vi "grub.vi"() -> ()   [LabVIEW 2014]
uses:
  <instrlib>/niDMM/nidmm.llb/niDMM Waveform Function.ctl
  <vilib>/Analysis/3filter.llb/Filter Passband Type.ctl
  <vilib>/Waveform/WDTOps.llb/WDT Get Waveform Subset DBL.vi
  <vilib>/Analysis/baseanly.llb/IIR Cascade Filter (DBL).vi
  <instrlib>/niDMM/nidmm.llb/niDMM Read Waveform (waveform data).vi
  <vilib>/Analysis/NI_AALBase.lvlib
  <vilib>/measure/NI_MABase.lvlib
  <vilib>/Analysis/NI_AALPro.lvlib
panel:
  in  "high cutoff freq: fh":dbl=0.45 format="%#_13g"
  out "DC estimate (V)":dbl caption="直流分量估计(V)" format="%0.2f"
  out "元素":waveform(dbl)
  in  "order":i32=2 caption="阶数"
  in  "low cutoff freq: fl":dbl=0.12500000000000006 caption="低截止频率:fl" format="%0.4f"
  out "波形图":ext[][](graph)
  out "Actual Number":i32
  in  "停止":bool
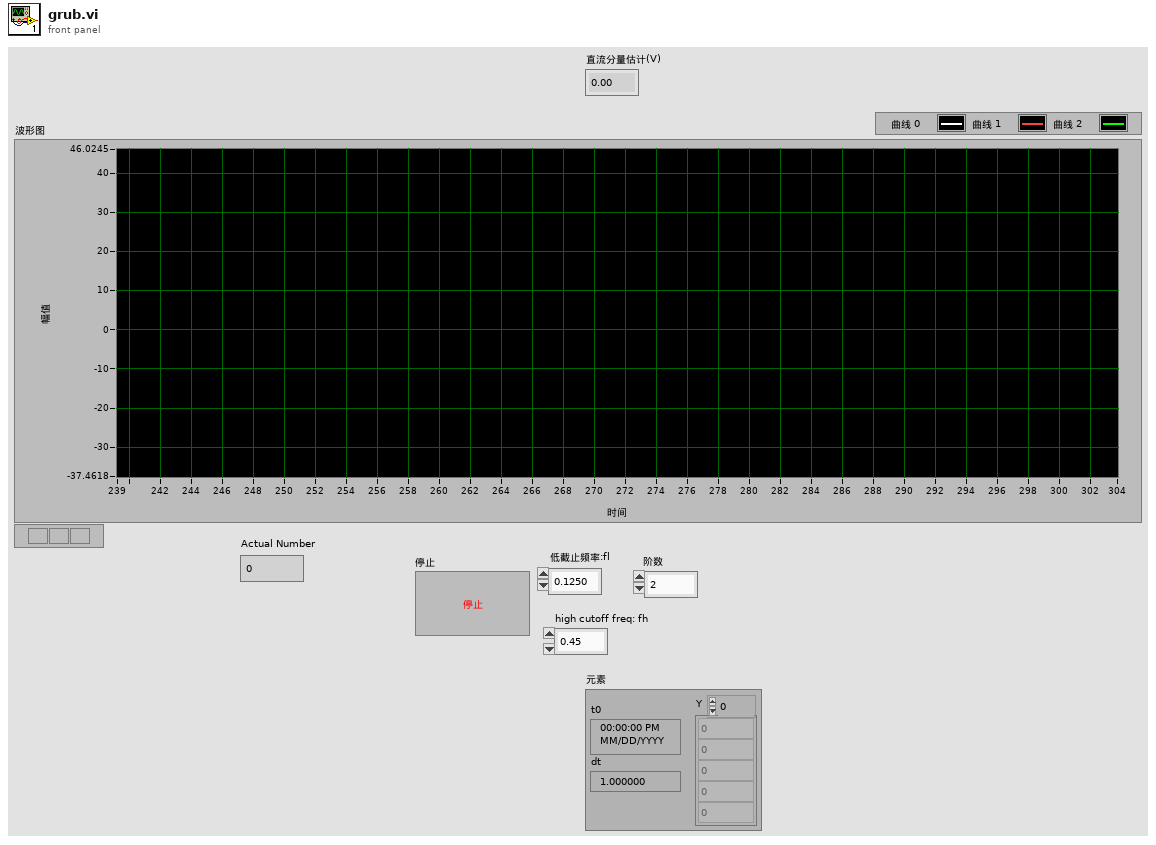
[diagram p1: front panel]
types:
  T1 = typedef "niDMM Waveform Function.ctl" = i32
  T2 = typedef "NI_AALBase.lvlib/Filter Passband Type.ctl" = enum32{"Lowpass", "Highpass", "Bandpass", "Bandstop"}
  T3 = cluster{"filter structure":enum32{"IIR 2nd Order", "IIR 4th Order"}, "Reverse Coefficients":dbl[], "Forward Coefficients":dbl[]}
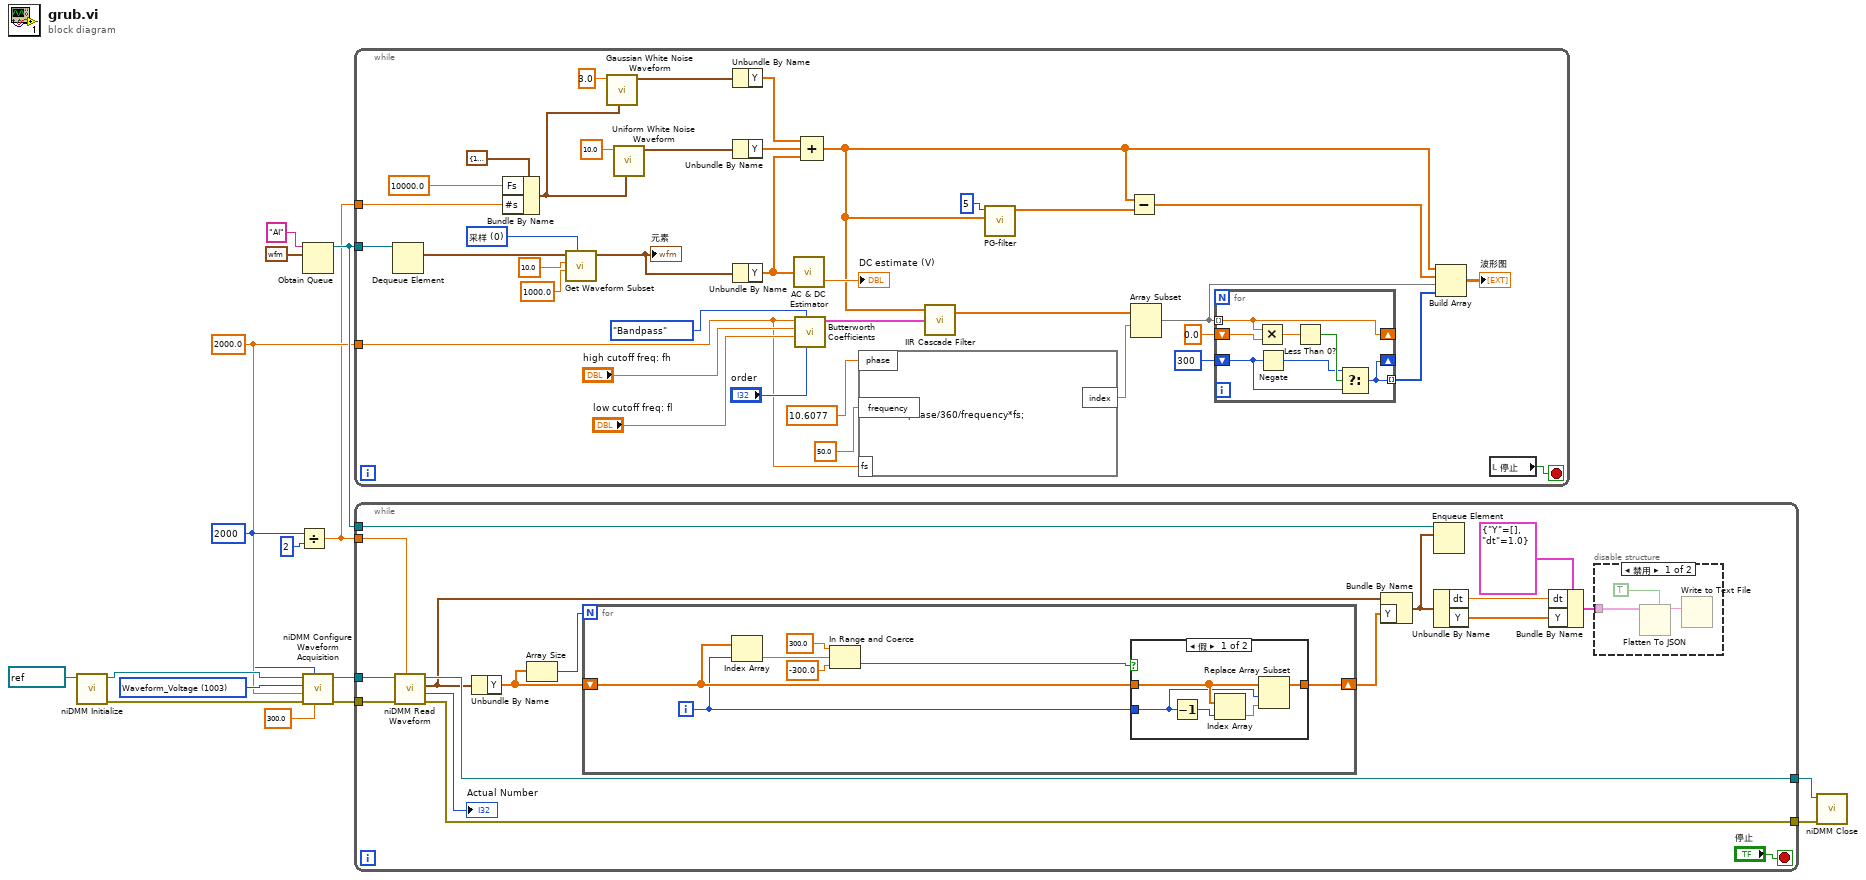
[diagram p0: block diagram]
diagram:
  w2 = 2000 ("Waveform Points")
  w4 = 2000.0 ("Rate")
  w16 = T1 1003 items=["Waveform_Voltage"=1003, "Waveform_Current"=1004] ("Function")
  n1 = call <instrlib>:"niDMM Initialize.vi"("Instrument Descriptor"=refnum<k15> "Dev1" ("instrument handle")) -> ("error out"=w13:errorcluster, "instrument handle out"=w14:refnum<k15>)  [unwired: 9 in]
  n2 = Divide(x=w2, y=2) -> (x/y=w1:dbl)
  n3 = Obtain Queue(name (unnamed)="AI" ("名称（未命名）"), element data type=waveform(dbl) {"t0"=timestamp(0 s since 1904-01-01), "dt"=1.0, "Y"=[]} ("输出波形")) -> (queue out=w5:refnum<queue>)  [unwired: 3 in, 2 out]
  n4 = call <instrlib>:"niDMM Configure Waveform Acquisition.vi"("Range"=300.0, "Waveform Points"=w2, "error in (no error)"=w13, "Rate"=w4, "Function"=w16, "instrument handle"=w14) -> ("error out"=w10:errorcluster, "instrument handle out"=w11:refnum<k15>)  [unwired: 4 in]
  n5 = while {
    tunnel: w5 -> [w53]
    tunnel: w4 -> [w22]
    tunnel: w1 -> [w43]
    stop <- w54 stop-if-true
    w30 = u16 0 items=["采样", "相对时间"] ("start/duration format")
    n6 = Dequeue Element(queue=w53) -> (element=w42:waveform(dbl))  [unwired: 2 in, 3 out]
    n7 = Bundle By Name(cluster=cluster{"Fs":dbl, "#s":dbl} {"Fs"=1000.0, "#s"=1000.0} ("sampling info"), "Fs"=10000.0, "#s"=w43) -> (w35:cluster{"Fs":dbl, "#s":dbl})
    n8 = call-poly <vilib>:"Get Waveform Subset.vi"("start/duration format"=w30, "duration"=1000.0, "start samples/time"=10.0, "waveform in"=w42) -> ("waveform out"=w32:waveform(dbl))  [unwired: 2 in, 3 out]
    "元素" <- w32
    n9 = call <vilib>:"Gaussian White Noise Waveform.vi"("sampling info"=w35, "standard deviation"=3.0) -> ("signal out"=w38:waveform(dbl))  [unwired: 8 in, 1 out]
    n10 = call <vilib>:"Uniform White Noise Waveform.vi"("sampling info"=w35, "amplitude"=10.0) -> ("signal out"=w41:waveform(dbl))  [unwired: 8 in, 1 out]
    n11 = Unbundle By Name(w38) -> ("Y"=w37:dbl[])
    n12 = Unbundle By Name(w41) -> ("Y"=w40:dbl[])
    n13 = Unbundle By Name(w32) -> ("Y"=w34:dbl[])
    n14 = call <vilib>:"AC & DC Estimator.vi"("Signal (V)"=w34) -> ("DC estimate (V)"=→"DC estimate (V)":dbl)  [unwired: 1 out]
    n15 = call <vilib>:"Butterworth Coefficients.vi"("order"="order", "filter type"=Filter_Passband_Type."Bandpass", "low cutoff freq: fl"="low cutoff freq: fl", "high cutoff freq: fh"="high cutoff freq: fh", "sampling freq: fs"=w22) -> ("IIR Filter Cluster"=w26:T3)  [unwired: 5 in, 1 out]
    n16 = Compound Arithmetic op=ADD(w37, w40, w34) -> (w27:dbl[])
    n17 = formula code="index = phase/360/frequency*fs;"("phase"=10.6077, "frequency"=50.0 ("输入变量"), "fs"=w22) -> ("index"=w21:dbl)
    n18 = call-poly <vilib>:"IIR Cascade Filter.vi"("IIR Filter Cluster"=w26, "X"=w27) -> ("Filtered X"=w25:dbl[])  [unwired: 1 in, 1 out]
    n19 = call "PG-filter.vi"("Y"=w27, "n"=i16 5) -> ("数组"=w52:ext[])  [unwired: 9 in]
    n20 = Subtract(x=w27, y=w52) -> (x-y=w49:ext[])
    n21 = Array Subset(array=w25, index=w21) -> (w20:dbl[])  [unwired: 1 in]
    n22 = for {
      tunnel: w20 -> [w59] mode=indexing
      shift-right: [w59] -> _
      shift-left: 0.0 -> [w61]
      shift-right: [w56] -> _
      shift-left: 300 -> [w57]
      tunnel: [w56] -> w17 mode=indexing
      n23 = Multiply(x=w59, y=w61) -> (x*y=w60:dbl)
      n24 = Negate(x=w57) -> (-x=w55:i32)
      n25 = Less Than 0?(x=w60) -> (x < 0?=w58:bool)
      n26 = Select(t=w55, s=w58, f=w57) -> (s? t:f=w56:i32)
    }
    n27 = Build Array(w27, w49, w20, w17) -> (→"波形图":ext[][])
    n28 = local read "停止"() -> (w54:bool)
  }
  n29 = while {
    tunnel: w11 -> [w78]
    tunnel: w10 -> [w77]
    tunnel: [w76] -> w9
    tunnel: [w75] -> w8
    tunnel: w5 -> [w64]
    tunnel: w1 -> [w62]
    stop <- "停止" stop-if-true
    n30 = call-poly <instrlib>:"niDMM Read Waveform.vi"("Number To Read"=w62, "error in (no error)"=w77, "instrument handle"=w78) -> ("error out"=w75:errorcluster, "Actual Number"=→"Actual Number":i32, "Waveform Data"=w73:waveform(dbl), "instrument handle out"=w76:refnum<k15>)  [unwired: 5 in]
    n31 = Unbundle By Name(w73) -> ("Y"=w71:dbl[])
    n32 = Array Size(array=w71) -> (size(s)=w70:i32)
    n33 = for {
      N: w70 -> [_]
      shift-right: [w88] -> w72
      shift-left: w71 -> [w84]
      i -> [w82]
      n34 = Index Array(array=w84, index=w82) -> (element=w83:dbl)
      n35 = In Range and Coerce(upper limit=300.0 ("上限"), x=w83, lower limit=-300.0 ("下限")) -> (In Range?=w85:bool)  [unwired: 1 out]
      n36 = case shown="假" w85 {
        tunnel: w84 -> [w92 w94]
        tunnel: [w91 w94] -> w88
        tunnel: w82 -> [w90 _]
        frame False {
          n37 = Decrement(x=w90) -> (x-1=w93:i32)
          n38 = Index Array(array=w92, index=w93) -> (element=w89:dbl)
          n39 = Replace Array Subset(array=w92, new element=w89, index=w90) -> (w91:dbl[])
        }
        frame True {
        }
      }
    }
    n40 = Bundle By Name(cluster=w73, "Y"=w72) -> (w63:waveform(dbl))
    n41 = Enqueue Element(queue=w64, element=w63) -> ()  [unwired: 2 in, 3 out]
    n42 = Unbundle By Name(w63) -> ("dt"=w67:dbl, "Y"=w66:dbl[])
    n43 = Bundle By Name(cluster=cluster{"Y":dbl[], "dt":dbl} {"Y"=[], "dt"=1.0} ("输入簇"), "dt"=w67, "Y"=w66) -> (w68:cluster{"Y":dbl[], "dt":dbl})
    n44 = disable-structure shown="禁用" {
      disable-tunnel: w68 -> [w80 _]
      frame Disabled {
        n45 = Flatten To JSON(enable LabVIEW extensions? (T)=TRUE ("启用LabVIEW扩展？(T)"), anything=w80) -> (JSON string=w79:string)  [unwired: 1 in, 1 out]
        n46 = Write to Text File(text=w79) -> ()  [unwired: 3 in, 3 out]
      }
      frame Enabled {
      }
    }
  }
  n47 = call <instrlib>:"niDMM Close.vi"("error in (no error)"=w8, "instrument handle"=w9) -> ()  [unwired: 9 in, 1 out]
